vi "ShooterSpeedRegulateV4.1.vi"(8 "Reset PID":bool, 11 "Shooter Speed":T1(ring)) -> (2 "Voltage Output":dbl, 3 "GO GO GO":bool)   [LabVIEW 2012]
uses:
  Robot Global Data.vi
panel:
  out "Motor Outputs":cluster{"Error":dbl, dbl, i32}(graph)
  out "Wheel 1 Setpoint":dbl
  out "Wheel 1 Error":dbl
  out "Wheel 1 Output":dbl
  out "Wheel 1 RPM":dbl
  # "SPEED Indexes            W1 Speed  |  W2 Speed\n0 - DEFAULT/OFF       0                     0\n1 - 2pt Shot                     21.25       9\n2 - 3pt Key Shot              24              14\n3 - Back Shot                     31.75       16.25\n4 - Fender Shot              15              7"
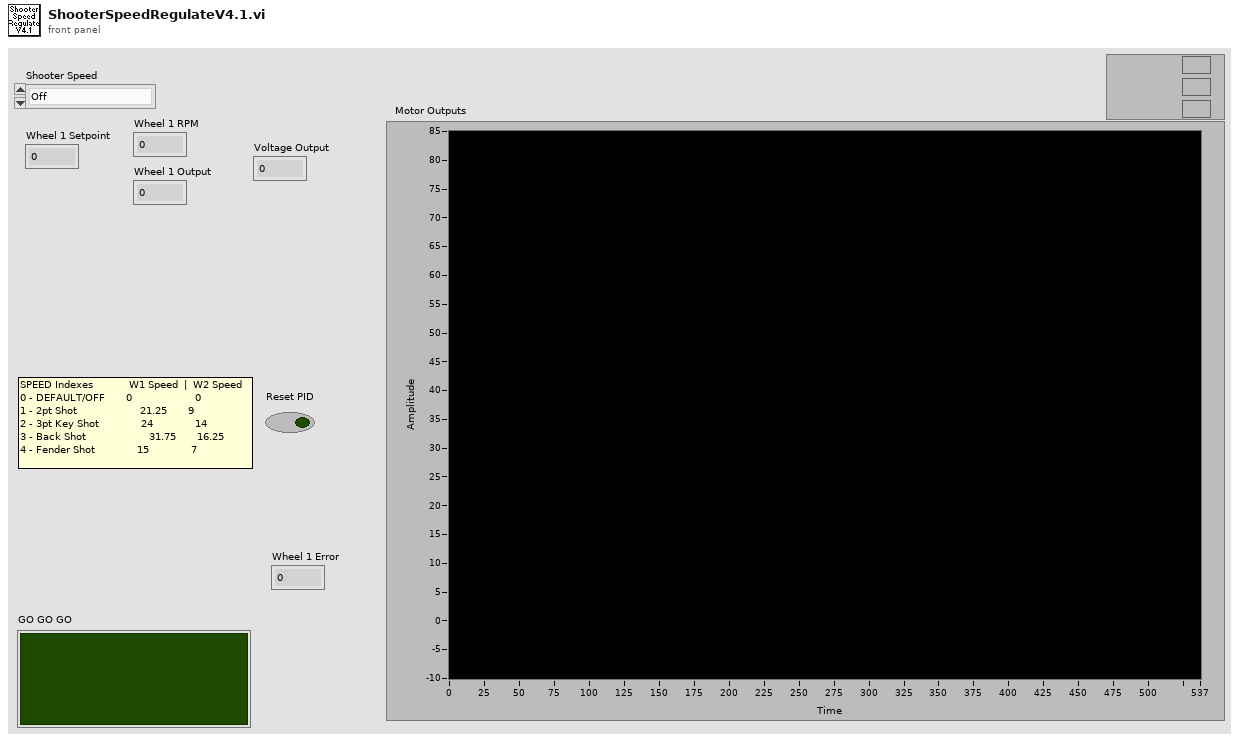
[diagram p1: front panel]
types:
  T1 = enum16{"Off", "Close Pyramid 3pt", "Far Pyramid 3pt", "Feeder Shot"}
  T2 = cluster{"proportional gain (Kc)":dbl, "integral time (Ti, min)":dbl, "derivative time (Td, min)":dbl}
  T3 = cluster{"Target Voltage":dbl, "Target Speed":dbl, "Angle Up?":bool}[]
  T4 = cluster{"Target Voltage":dbl, "Target Speed":dbl, "Angle Up?":bool}
  T5 = typedef "WPI_EncoderDevRef.ctl" = cluster{"DevStatus":errorcluster, "EncoderIndex":T6, "CounterIndex":T7, "DistancePerCount":dbl, "Decoding Type":T8}
  T6 = typedef "FPGA_EncoderIdx.ctl" = enum8{"Enc 0", "Enc 1", "Enc 2", "Enc 3", "Invalid"}
  T7 = typedef "FPGA_CounterCtrSystemIndex.ctl" = enum8{"Ctr 0", "Ctr 1", "Ctr 2", "Ctr 3", "Ctr 4", "Ctr 5", "Ctr 6", "Ctr 7", "Invalid"}
  T8 = typedef "WPI_EncoderType.ctl" = enum16{"1x", "2x", "4x"}
  T9 = cluster{"Wheel 1 PID-->Out":dbl, "Wheel 1 Out-->PID":dbl}
  T10 = typedef "WPI_MotorControlDeviceRef.ctl" = cluster{"DeviceStatus":errorcluster, "Type":enum16{"PWM", "CAN"}, "PWM":cluster{"Digital Module":T11, "PWM Channel":T12, "DeadBand":T13}, "CAN":cluster{"Device Number":u8, "Control Mode":T14, "Semaphore":T15, "Max Vout":dbl}, "Invert":bool, "TransformRef":T16, "InvTransformRef":T16}
  T11 = typedef "FPGA_TypedefDigitalModule.ctl" = enum16{"Digital Module 1", "Digital Module 2"}
  T12 = typedef "FPGA_DIOPWMChannel.ctl" = enum8{"PWM 1", "PWM 2", "PWM 3", "PWM 4", "PWM 5", "PWM 6", "PWM 7", "PWM 8", "PWM 9", "PWM 10", "Invalid"}
  T13 = typedef "WPI_PWMDeadband.ctl" = cluster{"Name":string, "maxPositivePwm":i32, "minPositivePwm":i32, "centerPwm":i32, "maxNegativePwm":i32, "minNegativePwm":i32, "angularRange":u16}
  T14 = typedef "WPI_CANJaguar_ControlMode.ctl" = enum8{"Percent VBus", "Current", "Speed", "Position", "Voltage"}
  T15 = typedef "Semaphore RefNum" = refnum<k1>
  T16 = typedef "WPI_PWMTransform_ConPane.ctl" = refnum<vi>
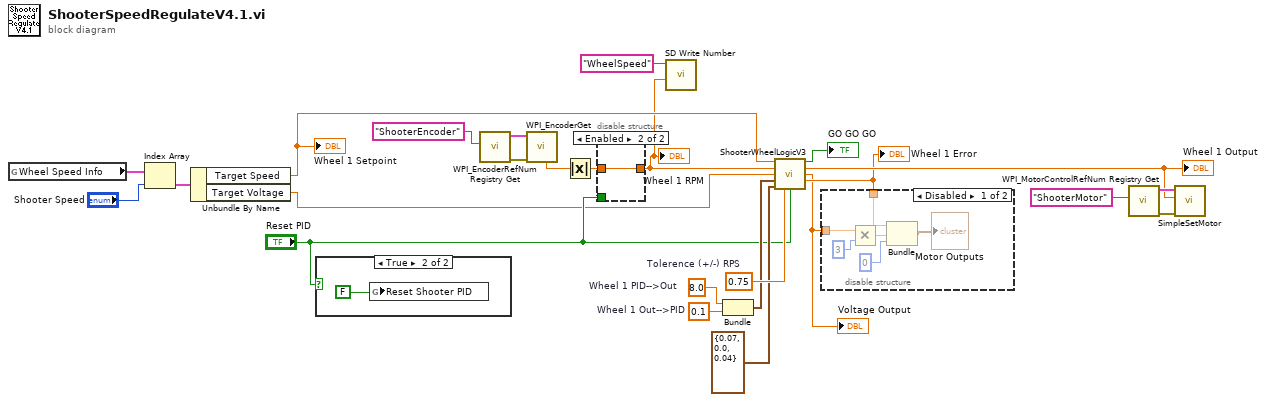
[diagram p0: block diagram]
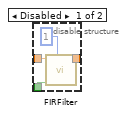
[diagram p3: hidden frame]
diagram:
  w17 = 0.1  # Wheel 1 Out-->PID
  w16 = 8.0  # Wheel 1 PID-->Out
  w24 = 0.75  # Tolerence (+/-) RPS
  n1 = global read "Robot Global Data.vi" "Wheel Speed Info"() -> (w10:T3)
  n2 = Index Array(array=w10, index="Shooter Speed") -> (element=w8:T4)
  n3 = Unbundle By Name(w8) -> ("Target Speed"=w4:dbl, "Target Voltage"=w7:dbl)
  "Wheel 1 Setpoint" <- w4
  n4 = case shown="True" "Reset PID" {
    frame False {
    }
    frame True {
      n5 = global write "Robot Global Data.vi" "Reset Shooter PID"(FALSE) -> ()
    }
  }
  n6 = call <vilib>:"WPI_EncoderRefNum Registry Get.vi"("refnum name"="ShooterEncoder") -> ("error out"=w13:errorcluster, "EncoderDevRef"=w14:T5)  [unwired: 9 in]
  n7 = call <vilib>:"WPI_EncoderGet.vi"("error in (no error)"=w13, "EncoderDevRef"=w14) -> ("Rate"=w12:dbl)  [unwired: 4 in, 5 out]
  n8 = Absolute Value(x=w12) -> (abs(x)=w11:dbl)
  n9 = disable-structure shown="Enabled" {
    disable-tunnel: "Reset PID" -> [w30 _]
    disable-tunnel: w11 -> [w29 w31]
    disable-tunnel: [w28 w31] -> w1
    frame Disabled {
      n10 = call "FIRFilter.vi"("Filter Size"=i8 1, "Reset"=w30, "Input"=w29) -> ("Output"=w28:dbl)  [unwired: 8 in]
    }
    frame Enabled {
    }
  }
  "Wheel 1 RPM" <- w1
  n11 = call <vilib>:"SD Write Number.vi"("Numeric"=w1, "Name"="WheelSpeed") -> ()  [unwired: 8 in, 2 out]
  n12 = Bundle("Wheel 1 PID-->Out"=w16, "Wheel 1 Out-->PID"=w17) -> (w20:T9)  [unwired: 1 in]
  n13 = call "ShooterWheelLogicV3.vi"("Setpoint"=w4, "Process Varaible"=w1, "Feedfoward Voltage"=w7, "SwitchZones"=w20, "PID gains"=T2 {"proportional gain (Kc)"=0.07, "integral time (Ti, min)"=0.0, "derivative time (Td, min)"=0.04} ("W1 PID gains"), "Error Margin"=w24, "Reset"="Reset PID") -> ("At Speed"=→"GO GO GO":bool, "Motor Output"=w21:dbl, "Voltage Output"=w5:dbl, "Error"=w6:dbl)  [unwired: 4 in, 1 out]
  "Wheel 1 Output" <- w21
  "Wheel 1 Error" <- w6
  "Voltage Output" <- w5
  n14 = disable-structure shown="Disabled" {
    disable-tunnel: w6 -> [w36 _]
    disable-tunnel: w5 -> [w32 _]
    frame Disabled {
      n15 = Multiply(x=w32, y=3) -> (x*y=w33:dbl)
      n16 = Bundle("Error"=w36, w33, 0) -> (→"Motor Outputs":cluster{"Error":dbl, dbl, i32})  [unwired: 1 in]
    }
    frame Enabled {
    }
  }
  n17 = call <vilib>:"WPI_MotorControlRefNum Registry Get.vi"("refnum name"="ShooterMotor") -> ("error out"=w22:errorcluster, "MotorControlDevRef"=w23:T10)  [unwired: 9 in]
  n18 = call "SimpleSetMotor.vi"("error in (no error)"=w22, "Output"=w21, "MotorControlDevRef"=w23) -> ()  [unwired: 7 in, 2 out]
